vi "ADS1015_Get_ADC_Value.vi"(5 "I2C Slave Address (0)":u8, 8 "error in (no error)":errorcluster, 9 "I2C_Channel_platform":T1, 10 "Scale Value (mV)":dbl=2.0, 11 "LINX Resource in":T2) -> (0 "error out":errorcluster, 2 "mV out":dbl, 3 "LINX Resource":T2, 4 "Data":u8[](array[numeric]))   [LabVIEW 2014]
uses:
  <vilib>/MakerHub/LINX/Private/Type Defs/LINX Ref.ctl
  <vilib>/MakerHub/LINX/Private/Type Defs/Platform.ctl
  <vilib>/MakerHub/LINX/Private/Type Defs/Interface.ctl
  <vilib>/MakerHub/LINX/Private/Device/Type Defs/LINX Device Config.ctl
  <vilib>/MakerHub/LINX/Private/Device/Type Defs/TCP Config.ctl
  <vilib>/MakerHub/LINX/Private/Device/Type Defs/Channels.ctl
  User Defined/I2C_Platform_Selector.ctl
  <vilib>/MakerHub/LINX/LMH-LINX.lvlib
  <vilib>/MakerHub/LINX/Private/Device/Device.lvlib
panel:
  out "(hi.lo)":u16
  out "16bit integer 3":i16
  out "16bit integer 2":i16 format="%.0b"
  out "16bit integer":i16 format="%.0b"
  in  "timespec":cluster{"sec":u32, "nsec":u32}
  in  "(hi.lo) 2":u16
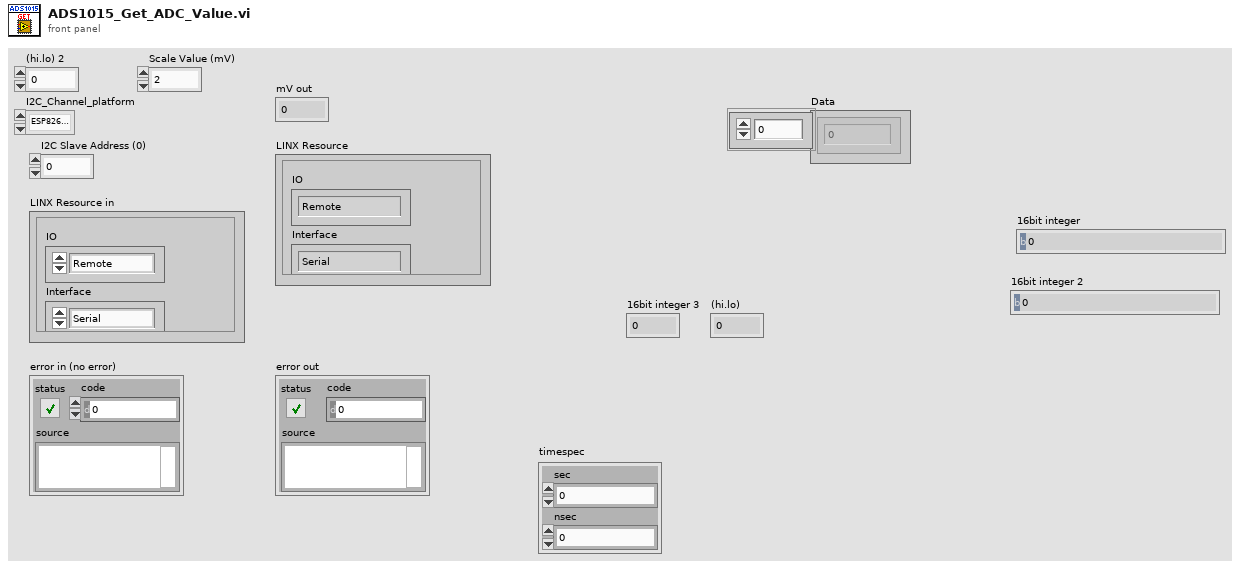
[diagram p1: front panel]
types:
  T1 = typedef "I2C_Platform_Selector.ctl" = enum16{"ESP8266-I2C", "Raspberry Pi-I2C"}
  T2 = typedef "LMH-LINX.lvlib/LINX Ref.ctl" = cluster{"IO":T3, "Interface":T4, "LINX Device Config":T5}
  T3 = typedef "LMH-LINX.lvlib/Platform.ctl" = enum16{"Remote", "Local"}
  T4 = typedef "LMH-LINX.lvlib/Interface.ctl" = enum16{"Serial", "TCP"}
  T5 = typedef "LMH-LINX.lvlib/Device.lvlib/LINX Device Config.ctl" = cluster{"Interface":T4, "COM Port":refnum<visa-resource-name>, "TCP Configuration":T6, "Device Family":u8, "Device ID":u8, "Device Name":string, "TCP Ref":refnum<k5>, "Channels":T7}
  T6 = typedef "LMH-LINX.lvlib/Device.lvlib/TCP Config.ctl" = cluster{"IP Address":string, "Port":u16}
  T7 = typedef "LMH-LINX.lvlib/Channels.ctl" = cluster{"DI":u8[], "DO":u8[], "AI":u8[], "AO":u8[], "PWM":u8[], "QE":u8[], "UART":u8[], "I2C 2":u8[], "SPI":u8[], "CAN":u8[], "Servo":u8[], "AI Ref (V)":dbl, "AI Resolution (Bits)":u8, "AO Ref (V)":dbl, "AO Resolution (Bits)":u8}
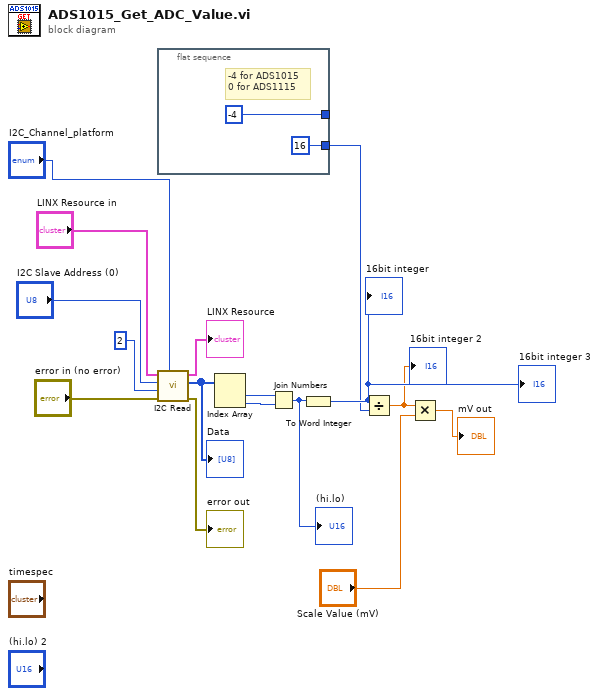
[diagram p0: block diagram]
diagram:
  n1 = flat-sequence {
    tunnel: [i8 -4 ("y")] -> _
    tunnel: [i16 16 ("y")] -> w2
    frame #0 {
      # "-4 for ADS1015 \n0 for ADS1115"
    }
  }
  n2 = call <vilib>:"I2C Read.vi"("I2C Channel"="I2C_Channel_platform", "Error In"="error in (no error)", "Bytes To Read"=u8 2, "I2C Slave Address (0)"="I2C Slave Address (0)", "LINX Resource"="LINX Resource in") -> ("Error Out"=→"error out":errorcluster, "Data"=w15:u8[], "LINX Resource"=→"LINX Resource":T2)  [unwired: 4 in]
  "Data" <- w15
  n3 = Index Array(array=w15) -> (element #1=w10:u8, element #2=w11:u8)  [unwired: 2 in]
  n4 = Join Numbers(hi=w10, lo=w11) -> ((hi.lo)=w4:u16)
  "(hi.lo)" <- w4
  n5 = To Word Integer(number=w4) -> (16bit integer=w3:i16)
  "16bit integer" <- w3
  "16bit integer 3" <- w3
  n6 = Divide(x=w3, y=w2) -> (x/y=w1:dbl)
  "16bit integer 2" <- w1
  n7 = Multiply(x=w1, y="Scale Value (mV)") -> (x*y=→"mV out":dbl)
